vi "Connect Multi Frame_BML.vi"(8 "error in (no error)":errorcluster, 10 "Timeset between frms":u32=50, 11 "BML Frame Array":refnum<class "BML_Frame_Root.lvclass">[](array[class])) -> (0 "error out":errorcluster, 3 "Connected Frame Contents":string)   [LabVIEW 2018, in "DigiPattern_Generator.lvclass"]
uses:
  DigiPattern_Generator.lvclass
  BML_Frame_Root/BML_Frame_Root.lvclass
  BML_Frame_Root/BML_Frame_Root.lvclass/BML_Frame_Root.ctl
  BML_Frame_Root/Special Frame.ctl
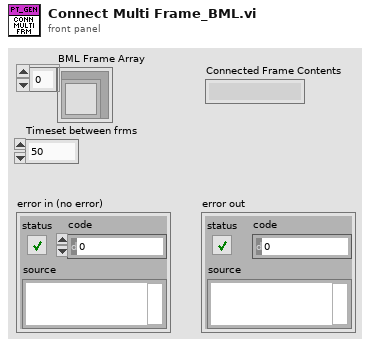
[diagram p1: front panel]
types:
  T1 = typedef "BML_Frame_Root.lvclass/Special Frame.ctl" = enum16{"Sync Header", "Protocol Header", "SW Trig", "SetID State", "Out SetID State", "SW Reset", "Wait", "SPI 4W FRM Start", "SPI 4W Wait", "SPI 4W FRM End", "SPI 4W Write Cmd", "SPI RD Collect Cmd", "SPI RD Value Cmd", "SPI 3W FRM Start", "SPI 3W Write Cmd", "SPI 3W FRM End", "SPI 3W Wait", "SPI 3W RD Cmd"}
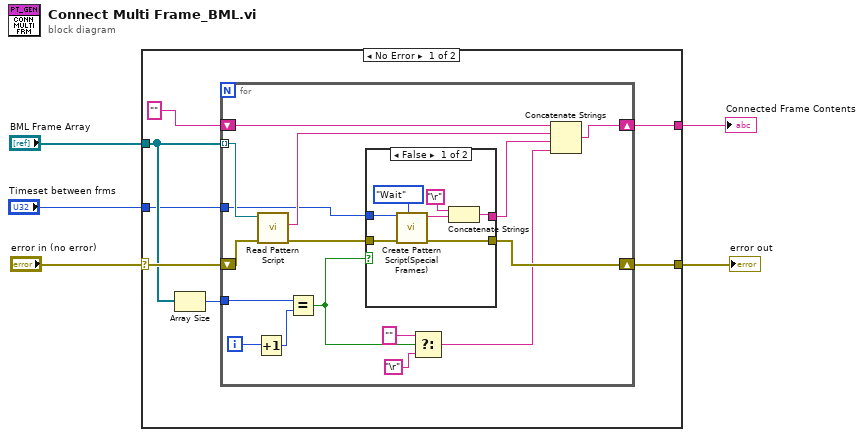
[diagram p0: block diagram]
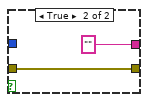
[diagram p2: hidden frame]
diagram:
  n1 = case shown="No Error" "error in (no error)" {
    selector: "error in (no error)" -> [w10 w38]
    tunnel: "BML Frame Array" -> [w9 _]
    tunnel: [w11 w38] -> w4
    tunnel: [w7 _] -> w2
    tunnel: "Timeset between frms" -> [w6 _]
    frame No Error {
      n2 = Array Size(array=w9) -> (size(s)=w8:i32)
      n3 = for {
        tunnel: w9 -> [w28] mode=indexing
        shift-right: [w18] -> w11
        shift-left: w10 -> [w27]
        shift-right: [w26] -> w7
        shift-left: "" -> [w25]
        tunnel: w8 -> [w17]
        tunnel: w6 -> [w13]
        i -> [w24]
        n4 = Increment(x=w24) -> (x+1=w23:i32)
        n5 = call "Read Pattern Script.vi"("error in (no error)"=w27, "BML_Frame_Root in"=w28) -> ("error out"=w19:errorcluster, "Pattern Script"=w16:string)  [unwired: 7 in, 1 out]
        n6 = Equal?(x=w17, y=w23) -> (x = y?=w20:bool)
        n7 = case shown="False" w20 {
          tunnel: w19 -> [w35 w36]
          tunnel: [w34 w36] -> w18
          tunnel: w13 -> [w33 _]
          tunnel: [w30 "" ("string out")] -> w14
          frame False {
            n8 = call "Create Pattern Script(Special Frames).vi"("Special Frame Type"=Special_Frame."Wait", "error in (no error)"=w35, "Num of Timeset"=w33) -> ("error out"=w34:errorcluster, "string out"=w31:string)  [unwired: 7 in]
            n9 = Concatenate Strings("\r", w31) -> (w30:string)
          }
          frame True {
          }
        }
        n10 = Select(t="", s=w20, f="\r") -> (s? t:f=w15:string)
        n11 = Concatenate Strings(w25, w16, w14, w15) -> (w26:string)
      }
    }
    frame Error {
    }
  }
  "error out" <- w4
  "Connected Frame Contents" <- w2
